vi "Initialize.vi"(8 "Error In":errorcluster, 11 "VISA in":refnum<visa-resource-name>) -> (0 "Error Out":errorcluster)   [LabVIEW 2019, in "Allmotion.lvlib"]
uses:
  Allmotion.lvlib
  Queues/Queues.lvlib
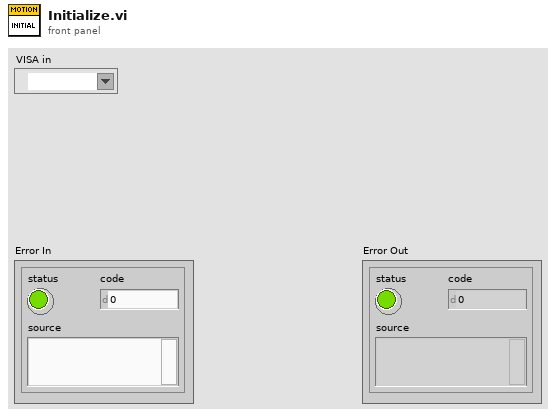
[diagram p1: front panel]
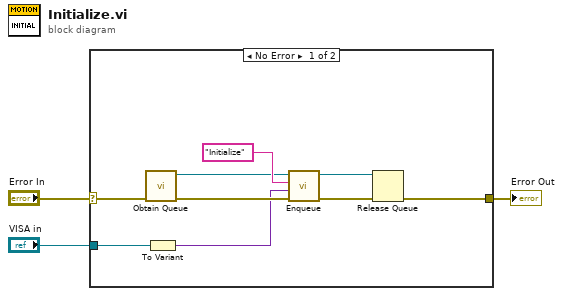
[diagram p0: block diagram]
diagram:
  n1 = case shown="No Error" "Error In" {
    selector: "Error In" -> [w11 w13]
    tunnel: [w7 w13] -> w3
    tunnel: "VISA in" -> [w5 _]
    frame No Error {
      n2 = call "Obtain Queue.vi"("Error In"=w11) -> ("Error Out"=w10:errorcluster, "Queue out"=w9:refnum<queue>)  [unwired: 9 in]
      n3 = To Variant(anything=w5) -> (Variant=w4:variant)
      n4 = call "Enqueue.vi"("Error In"=w10, "Data"=w4, "State"="Initialize", "Queue in"=w9) -> ("Error Out"=w8:errorcluster, "Queue out"=w6:refnum<queue>)  [unwired: 6 in]
      n5 = Release Queue(queue=w6, error in (no error)=w8) -> (error out=w7:errorcluster)  [unwired: 1 in, 2 out]
    }
    frame Error {
    }
  }
  "Error Out" <- w3
